vi "Move Bullets.vi"(8 "error in (no error)":errorcluster, 11 "Game Data in":T1) -> (0 "error out":errorcluster, 3 "Game Data out":T1)   [LabVIEW 2025]
uses:
  Game Data.ctl
  Bullet Data.ctl
  Game State.ctl
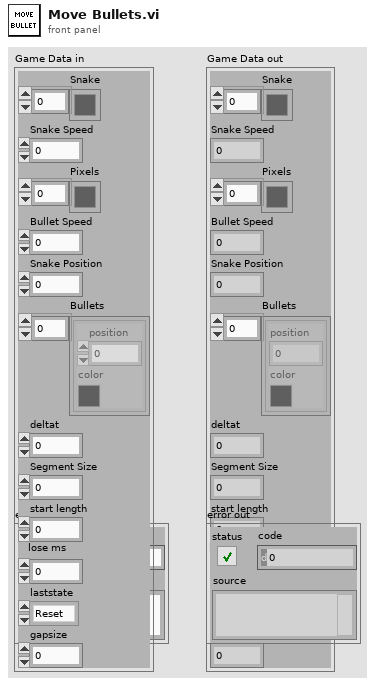
[diagram p1: front panel]
types:
  T1 = typedef "Game Data.ctl" = cluster{"Snake":u32[], "Snake Speed":dbl, "Pixels":u32[], "Bullet Speed":dbl, "Snake Position":dbl, "Bullets":T2[], "deltat":dbl, "Segment Size":dbl, "start length":u32, "lose ms":u32, "laststate":T3, "gapsize":i32}
  T2 = typedef "Bullet Data.ctl" = cluster{"position":dbl, "color":u32}
  T3 = typedef "Game State.ctl" = enum16{"Reset", "Idle", "Start", "Playing", "Win", "Lose"}
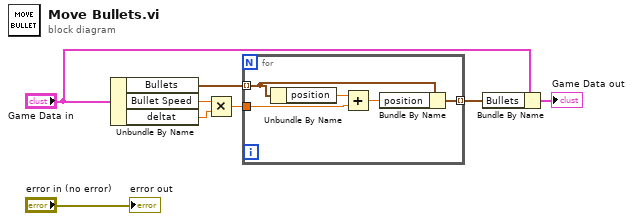
[diagram p0: block diagram]
diagram:
  n1 = Unbundle By Name("Game Data in") -> ("Bullets"=w5:T2[], "Bullet Speed"=w4:dbl, "deltat"=w3:dbl)
  n2 = Multiply(x=w4, y=w3) -> (x*y=w2:dbl)
  n3 = for {
    tunnel: w5 -> [w11] mode=indexing
    tunnel: w2 -> [w12]
    tunnel: [w9] -> w1 mode=indexing
    n4 = Unbundle By Name(w11) -> ("position"=w13:dbl)
    n5 = Add(x=w13, y=w12) -> (x+y=w10:dbl)
    n6 = Bundle By Name(cluster=w11, "position"=w10) -> (w9:T2)
  }
  n7 = Bundle By Name(cluster="Game Data in", "Bullets"=w1) -> (→"Game Data out":T1)
  "error out" <- "error in (no error)"
